vi "Refresh Available Resources(High Level).vi"(5 "Filter Names":string[](array[string]), 7 "Filter Type":T1=enum."Product Name", 8 "error in (no error)":errorcluster, 11 "Section Ref in":T2 format="%.0x") -> (0 "error out":errorcluster, 1 "Name and Alias":string[](array[string]), 2 "Aliases":string[](array[string]), 3 "Section Ref out":T2=18446744073709551615 format="%.0x")   [LabVIEW 2019, in "NIVS Hardware Discovery.lvlib"]
uses:
  NIVS Hardware Discovery.lvlib
  <vilib>/NI VeriStand/Custom Device API/Custom Device Item Ref.ctl
  _Types/Filter Type.ctl
  <vilib>/NI VeriStand/Custom Device API/Custom Device API.lvlib
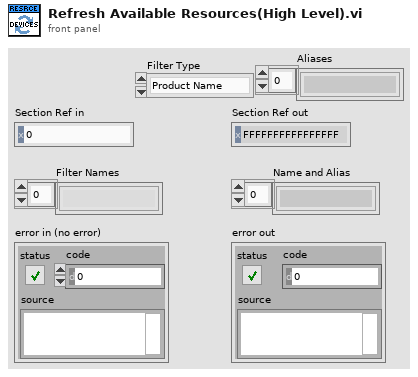
[diagram p1: front panel]
types:
  T1 = typedef "NIVS Hardware Discovery.lvlib/Filter Type.ctl" = enum16{"Device Category", "Product Name", "Ethernet", "XNET", "VISA", "FPGA", "EtherCAT Master", "DAQmx", "GPIB", "Serial"}
  T2 = typedef "Custom Device API.lvlib/Custom Device Item Ref.ctl" = u64
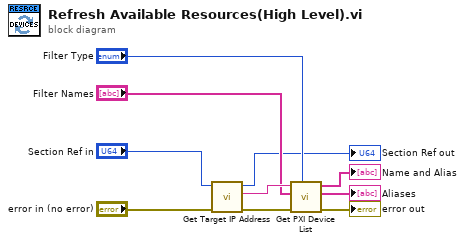
[diagram p0: block diagram]
diagram:
  n1 = call "Get Target IP Address.vi"("error in"="error in (no error)", "Device Item Ref in"="Section Ref in") -> ("error out"=w7:errorcluster, "IP Address"=w10:string, "Device Item Ref out"=→"Section Ref out":T2)  [unwired: 7 in]
  n2 = call "Get PXI Device List.vi"("Filter Type"="Filter Type", "error in (no error)"=w7, "Filter Names"="Filter Names", "Target IP Address"=w10) -> ("error out"=→"error out":errorcluster, "Alias"=→"Aliases":string[], "Name and Alias"=→"Name and Alias":string[])  [unwired: 5 in]
